vi "TraceLoggerSnapshotBroadcast_Parse.vi"(8 "error in (no error)":errorcluster, 11 "MsgValue":variant) -> (0 "error out":errorcluster, 3 "TraceLoggerSnapshotBroadcast":T1)   [LabVIEW 2017, in "TracePointSynchronizer.lvlib"]
uses:
  <vilib>/addons/InsightCM/Devices/Shared/Common/TracePointSynchronizer/TracePointSynchronizer.lvlib
  <vilib>/addons/InsightCM/MessageBus/MessageLibrary/TraceLogger/controls/TraceLoggerSnapshotBroadcast.ctl
  <vilib>/addons/InsightCM/MessageBus/Base/controls/MessageHeader.ctl
  <vilib>/addons/InsightCM/MessageBus/Base/controls/KeyValuePair.ctl
  <vilib>/addons/InsightCM/MessageBus/MessageLibrary/TraceLogger/controls/TraceLoggerSnapshotBroadcastBody.ctl
  <vilib>/addons/InsightCM/MessageBus/Base/controls/TracePointSetting.ctl
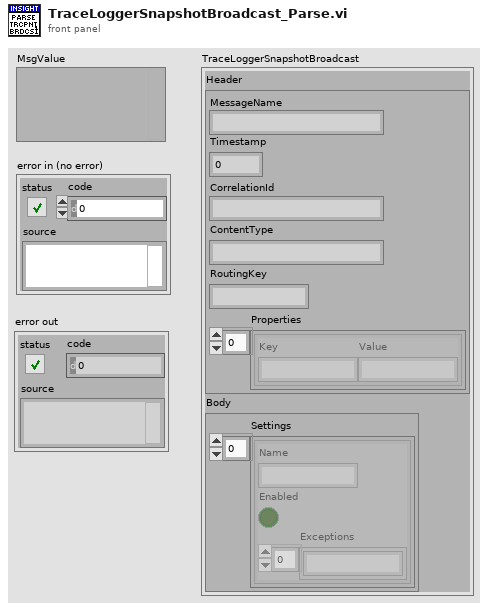
[diagram p1: front panel]
types:
  T1 = typedef "TraceLoggerSnapshotBroadcast.ctl" = cluster{"Header":T2, "Body":T4}
  T2 = typedef "MessageHeader.ctl" = cluster{"MessageName":string, "Timestamp":i64, "CorrelationId":string, "ContentType":string, "RoutingKey":string, "Properties":T3[]}
  T3 = typedef "KeyValuePair.ctl" = cluster{"Key":string, "Value":string}
  T4 = typedef "TraceLoggerSnapshotBroadcastBody.ctl" = cluster{"Settings":T5[]}
  T5 = typedef "TracePointSetting.ctl" = cluster{"Name":string, "Enabled":bool, "Exceptions":string[]}
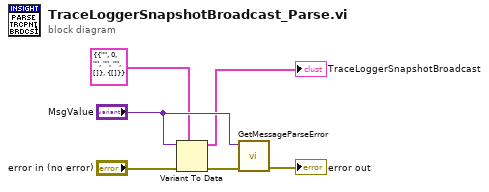
[diagram p0: block diagram]
diagram:
  n1 = Variant To Data(error in="error in (no error)", type=T1 {"Header"={"MessageName"="", "Timestamp"=0, "CorrelationId"="", "ContentType"="", "RoutingKey"="", "Properties"=[]}, "Body"={"Settings"=[]}} ("TraceLoggerSnapshotBroadcast"), Variant="MsgValue") -> (data=→"TraceLoggerSnapshotBroadcast":T1, error out=w6:errorcluster)
  n2 = call <vilib>:"GetMessageParseError.vi"("error in (no error)"=w6, "body"="MsgValue") -> ("error out"=→"error out":errorcluster)  [unwired: 7 in, 2 out]
